vi "Set Weave Lift Motor Output.vi"(3 "Output":dbl) -> (0 "Upper Switch Pressed":bool, 1 "Lower Switch Pressed":bool, 2 "Motor Value":dbl)   [LabVIEW 2015]
uses:
  Robot Global Data.vi
  <vilib>/Rock Robotics/Network Tables/NT Write Number.vi
panel:
  in  "Upper Switch":bool
  in  "Lower Switch":bool
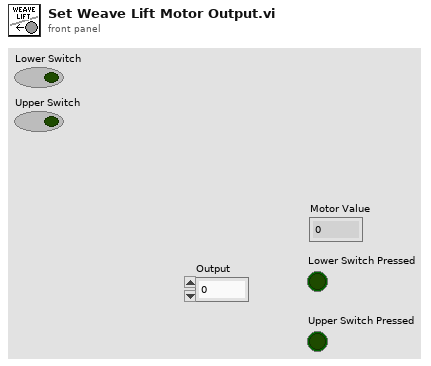
[diagram p1: front panel]
types:
  T1 = typedef "WPI_SwitchDevRef.ctl" = cluster{"DevStatus":errorcluster, "DIO Channel":T2, "CntIndex":T3, "Normally Closed":bool}
  T2 = typedef "FPGA_DIOChannel.ctl" = enum8{"DIO 0", "DIO 1", "DIO 2", "DIO 3", "DIO 4", "DIO 5", "DIO 6", "DIO 7", "DIO 8", "DIO 9", "DIO MXP 0", "DIO MXP 1", "DIO MXP 2", "DIO MXP 3", "DIO MXP 4", "DIO MXP 5", "DIO MXP 6", "DIO MXP 7", "DIO MXP 8", "DIO MXP 9", "DIO MXP 10", "DIO MXP 11", "DIO MXP 12", "DIO MXP 13", "DIO MXP 14", "DIO MXP 15", "Invalid"}
  T3 = typedef "FPGA_CounterCtrSystemIndex.ctl" = enum8{"Ctr 0", "Ctr 1", "Ctr 2", "Ctr 3", "Ctr 4", "Ctr 5", "Ctr 6", "Ctr 7", "Invalid"}
  T4 = typedef "WPI_MotorControlDeviceRef.ctl" = cluster{"DeviceStatus":errorcluster, "Type":T5, "PWM":cluster{"PWM Channel":T6, "DeadBand":T7}, "CAN":cluster{"Device Number":u8, "Control Mode":T8, "Semaphore":T9, "Max Vout":dbl, "TalonSRX Control Mode":T10}, "Invert":bool}
  T5 = typedef "WPI_MotorControlType.ctl" = enum16{"PWM", "CAN", "CANTalonSRX"}
  T6 = typedef "FPGA_DIOPWMChannel.ctl" = enum8{"PWM 0", "PWM 1", "PWM 2", "PWM 3", "PWM 4", "PWM 5", "PWM 6", "PWM 7", "PWM 8", "PWM 9", "PWM MXP 0", "PWM MXP 1", "PWM MXP 2", "PWM MXP 3", "PWM MXP 4", "PWM MXP 5", "PWM MXP 6", "PWM MXP 7", "PWM MXP 8", "PWM MXP 9", "Invalid"}
  T7 = typedef "WPI_PWMDeadband.ctl" = cluster{"Name":string, "maxPositivePwm":i32, "minPositivePwm":i32, "centerPwm":i32, "maxNegativePwm":i32, "minNegativePwm":i32, "angularRange":u16}
  T8 = typedef "WPI_CANJaguar_ControlMode.ctl" = enum8{"Percent VBus", "Current", "Speed", "Position", "Voltage"}
  T9 = typedef "Semaphore RefNum" = refnum<k1>
  T10 = typedef "WPI_CANTalonSRX_APIControlMode.ctl" = enum8{"Percent VBus", "Speed", "Position", "Slave", "Unchanged / Invalid", "Voltage Compensation", "Current", "Motion Profile"}
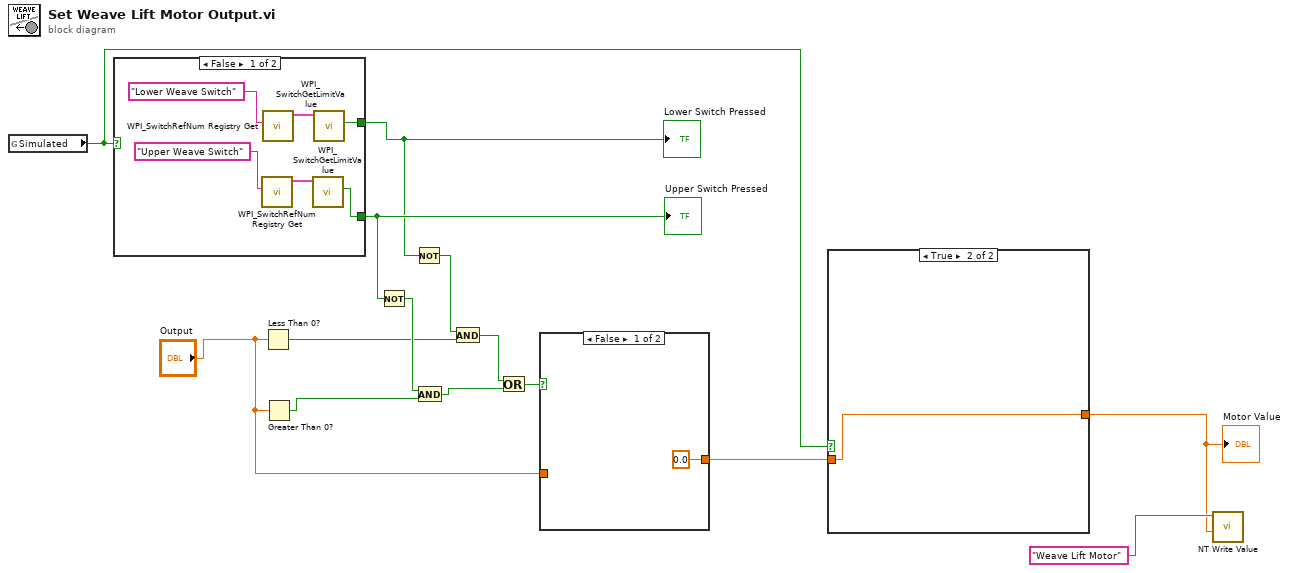
[diagram p0: block diagram]
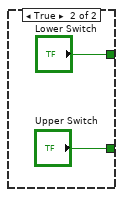
[diagram p2: hidden frame]
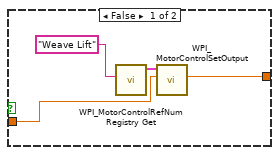
[diagram p3: hidden frame]
diagram:
  n1 = global read "Robot Global Data.vi" "Simulated"() -> (w3:bool)
  n2 = case shown="False" w3 {
    tunnel: [w16 "Upper Switch"] -> w13
    tunnel: [w15 "Lower Switch"] -> w10
    frame False {
      n3 = call <vilib>:"WPI_SwitchRefNum Registry Get.vi"("refnum name"="Upper Weave Switch") -> ("SwitchDevRef"=w17:T1)  [unwired: 9 in, 1 out]
      n4 = call <vilib>:"WPI_SwitchRefNum Registry Get.vi"("refnum name"="Lower Weave Switch") -> ("SwitchDevRef"=w18:T1)  [unwired: 9 in, 1 out]
      n5 = call <vilib>:"WPI_SwitchGetLimitValue.vi"("SwitchDevRef"=w17) -> ("Switch Pressed"=w16:bool)  [unwired: 8 in, 2 out]
      n6 = call <vilib>:"WPI_SwitchGetLimitValue.vi"("SwitchDevRef"=w18) -> ("Switch Pressed"=w15:bool)  [unwired: 8 in, 2 out]
    }
    frame True {
    }
  }
  "Lower Switch Pressed" <- w10
  "Upper Switch Pressed" <- w13
  n7 = Less Than 0?(x="Output") -> (x < 0?=w8:bool)
  n8 = Greater Than 0?(x="Output") -> (x > 0?=w12:bool)
  n9 = Not(x=w13) -> (.not. x?=w11:bool)
  n10 = Not(x=w10) -> (.not. x?=w9:bool)
  n11 = And(x=w11, y=w12) -> (x .and. y?=w6:bool)
  n12 = And(x=w9, y=w8) -> (x .and. y?=w7:bool)
  n13 = Or(x=w7, y=w6) -> (x .or. y?=w14:bool)
  n14 = case shown="False" w14 {
    tunnel: "Output" -> [_ w24]
    tunnel: [0.0 ("Output") w24] -> w4
    frame False {
    }
    frame True {
    }
  }
  n15 = case shown="True" w3 {
    tunnel: w4 -> [w27 w29]
    tunnel: [w25 w29] -> w1
    frame False {
      n16 = call <vilib>:"WPI_MotorControlRefNum Registry Get.vi"("refnum name"="Weave Lift") -> ("MotorControlDevRef"=w28:T4)  [unwired: 9 in, 1 out]
      n17 = call <vilib>:"WPI_MotorControlSetOutput.vi"("Output"=w27, "MotorControlDevRef"=w28) -> ("Motor Output"=w25:dbl)  [unwired: 7 in, 2 out]
    }
    frame True {
    }
  }
  "Motor Value" <- w1
  n18 = call-poly <vilib>:"NT Write Value.vi"("Numeric"=w1, "Name"="Weave Lift Motor") -> ()  [unwired: 9 in, 1 out]
